vi "fgv_Sys Config.vi"(8 "error in (no error)":errorcluster, 10 "Function":T11, 11 "System Config in":T1={"XY Stage"={"COM port"="", "XY stage available"=FALSE}, "DAQ FPGA"={"Ref"=refnum, "Target"="RIO0", "Clock Freq (MHz) "=200.0, "input card type"=enum."AC Card", "Samples Wait after Trigger"=5080, "AOD fill"=4900, "StartupDelay"=0, "Slip Cycle (clock cycles)"=600000, "Add Cycle"=TRUE}, "Control system"={"Ethernet opened"=FALSE, "Ethernet Port"=3, "Ctrl FPGA available"=FALSE, "Ctrl FPGA Clock (MHz)"=240.0, "Ctrl system MAC address"="", "Control system.Network adapter name"="", "AOD 1 Amplitude"=0, "AOD 2 Amplitude"=0, "AOD 3 Amplitude"=0, "AOD 4 Amplitude"=0, "Data Time Interval (ns)"=0.0, "T0 (ns)"=0.0, "Ta (ns)"=0.0}, "Encoder"={"IP address"="224.0.1.103", "Port"=7000, "Encoder available"=FALSE, "Wheel radius (cm)"=16.0}, "DAQmx Chan"={"Pockels AO"="", "Hard shutter AO"="", "PMT AOs"="", "Power meter AI"=""}, "Computer MAC address"="", "Cam VidRec"={"DO flag-Video record"="", "DO flag-Trial start"="", "VidRec available"=FALSE}, "Externalise Triggers"=FALSE, "Laser wavelength (nm)"=920.0} {"Laser wavelength (nm)" min=800.0 max=1080.0 step=1.0; "Encoder"."Wheel radius (cm)" format="%#_13g"; "Control system"."Ctrl FPGA Clock (MHz)" min=80.0 max=500.0 step=1.0; "Control system"."Data Time Interval (ns)" min=0.0 max=2048.0 step=1.0; "Control system"."Ta (ns)" min=0.0 max=2048.0 step=1.0; "Control system"."T0 (ns)" min=0.0 max=2048.0 step=1.0; "Control system"."AOD 4 Amplitude" min=0 max=2048 step=1; "Control system"."AOD 3 Amplitude" min=0 max=2048 step=1; "Control system"."AOD 2 Amplitude" min=0 max=2048 step=1; "Control system"."AOD 1 Amplitude" min=0 max=2048 step=1}) -> (0 "error out":errorcluster, 3 "System Config out":T1={"XY Stage"={"COM port"="", "XY stage available"=FALSE}, "DAQ FPGA"={"Ref"=refnum, "Target"="RIO0", "Clock Freq (MHz) "=200.0, "input card type"=enum."AC Card", "Samples Wait after Trigger"=5080, "AOD fill"=4900, "StartupDelay"=0, "Slip Cycle (clock cycles)"=600000, "Add Cycle"=TRUE}, "Control system"={"Ethernet opened"=FALSE, "Ethernet Port"=3, "Ctrl FPGA available"=FALSE, "Ctrl FPGA Clock (MHz)"=240.0, "Ctrl system MAC address"="", "Control system.Network adapter name"="", "AOD 1 Amplitude"=0, "AOD 2 Amplitude"=0, "AOD 3 Amplitude"=0, "AOD 4 Amplitude"=0, "Data Time Interval (ns)"=0.0, "T0 (ns)"=0.0, "Ta (ns)"=0.0}, "Encoder"={"IP address"="224.0.1.103", "Port"=7000, "Encoder available"=FALSE, "Wheel radius (cm)"=16.0}, "DAQmx Chan"={"Pockels AO"="", "Hard shutter AO"="", "PMT AOs"="", "Power meter AI"=""}, "Computer MAC address"="", "Cam VidRec"={"DO flag-Video record"="", "DO flag-Trial start"="", "VidRec available"=FALSE}, "Externalise Triggers"=FALSE, "Laser wavelength (nm)"=920.0} {"Laser wavelength (nm)" min=800.0 max=1080.0 step=1.0; "Encoder"."Wheel radius (cm)" format="%#_13g"; "Control system"."Ctrl FPGA Clock (MHz)" min=80.0 max=500.0 step=1.0; "Control system"."Data Time Interval (ns)" min=0.0 max=2048.0 step=1.0; "Control system"."Ta (ns)" min=0.0 max=2048.0 step=1.0; "Control system"."T0 (ns)" min=0.0 max=2048.0 step=1.0; "Control system"."AOD 4 Amplitude" min=0 max=2048 step=1; "Control system"."AOD 3 Amplitude" min=0 max=2048 step=1; "Control system"."AOD 2 Amplitude" min=0 max=2048 step=1; "Control system"."AOD 1 Amplitude" min=0 max=2048 step=1})   [LabVIEW 2013]
uses:
  Typedefs/Sys Configuration.ctl
  Typedefs/XY Stage config cluster.ctl
  Typedefs/DAQ FPGA config cluster.ctl
  RIG-SPECIFIC FILES/FPGA Refs/FPGA Ref.ctl
  <vilib>/userdefined/High Color/nirio_resource_hc.ctl
  Typedefs/FPGA input type AC-DC.ctl
  Typedefs/CTRL system config cluster.ctl
  Typedefs/Encoder config cluster.ctl
  Typedefs/DAQmx physical channels cluster.ctl
  Typedefs/Cam VidRec HW config setup cluster.ctl
  Typedefs/HW config states enum.ctl
  Typedefs/Save-Load enum.ctl
panel:
  # "FUNCTIONAL GLOBAL"
  # "<--- The \"PMT AOs\" DAQmx string will always contain\n                       2 channels is this format: PXI1Slot4/ao2:3"
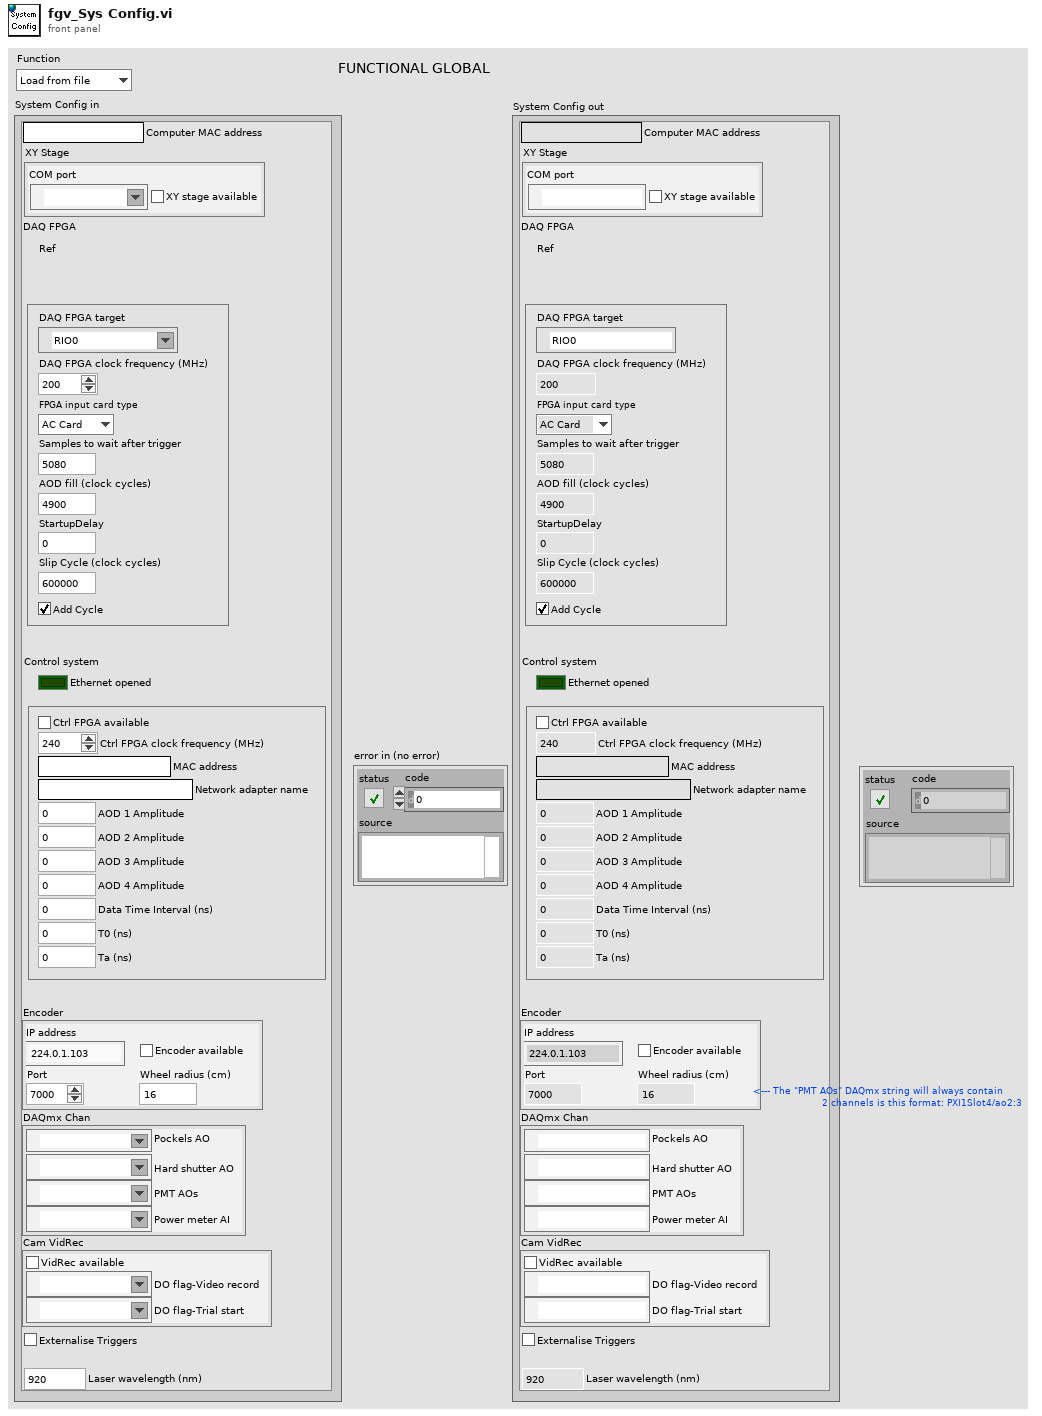
[diagram p1: front panel]
types:
  T1 = typedef "Sys Configuration.ctl" = cluster{"XY Stage":T2, "DAQ FPGA":T3, "Control system":T7, "Encoder":T8, "DAQmx Chan":T9, "Computer MAC address":string, "Cam VidRec":T10, "Externalise Triggers":bool, "Laser wavelength (nm)":dbl}
  T2 = typedef "XY Stage config cluster.ctl" = cluster{"COM port":refnum<visa-resource-name>, "XY stage available":bool}
  T3 = typedef "DAQ FPGA config cluster.ctl" = cluster{"Ref":T4, "Target":T5, "Clock Freq (MHz) ":dbl, "input card type":T6, "Samples Wait after Trigger":u16, "AOD fill":u16, "StartupDelay":i32, "Slip Cycle (clock cycles)":u32, "Add Cycle":bool}
  T4 = typedef "FPGA Ref.ctl" = refnum<k20>
  T5 = typedef "nirio_resource_hc.ctl" = tag
  T6 = typedef "FPGA input type AC-DC.ctl" = enum16{"AC Card", "DC Card"}
  T7 = typedef "CTRL system config cluster.ctl" = cluster{"Ethernet opened":bool, "Ethernet Port":u32, "Ctrl FPGA available":bool, "Ctrl FPGA Clock (MHz)":dbl, "Ctrl system MAC address":string, "Control system.Network adapter name":string, "AOD 1 Amplitude":i16, "AOD 2 Amplitude":i16, "AOD 3 Amplitude":i16, "AOD 4 Amplitude":i16, "Data Time Interval (ns)":dbl, "T0 (ns)":dbl, "Ta (ns)":dbl}
  T8 = typedef "Encoder config cluster.ctl" = cluster{"IP address":string, "Port":u16, "Encoder available":bool, "Wheel radius (cm)":dbl}
  T9 = typedef "DAQmx physical channels cluster.ctl" = cluster{"Pockels AO":tag, "Hard shutter AO":tag, "PMT AOs":tag, "Power meter AI":tag}
  T10 = typedef "Cam VidRec HW config setup cluster.ctl" = cluster{"DO flag-Video record":tag, "DO flag-Trial start":tag, "VidRec available":bool}
  T11 = typedef "HW config states enum.ctl" = enum16{"Load from file", "Save to file", "Write all", "Read all", "Write XY stage settings", "Write DAQ FPGA settings", "Write Control FPGA settings", "Write Phys Channels", "Clear", "Compare from file"}
  T12 = typedef "Save-Load enum.ctl" = enum16{"Save to file", "Load from file", "Compare from file"}
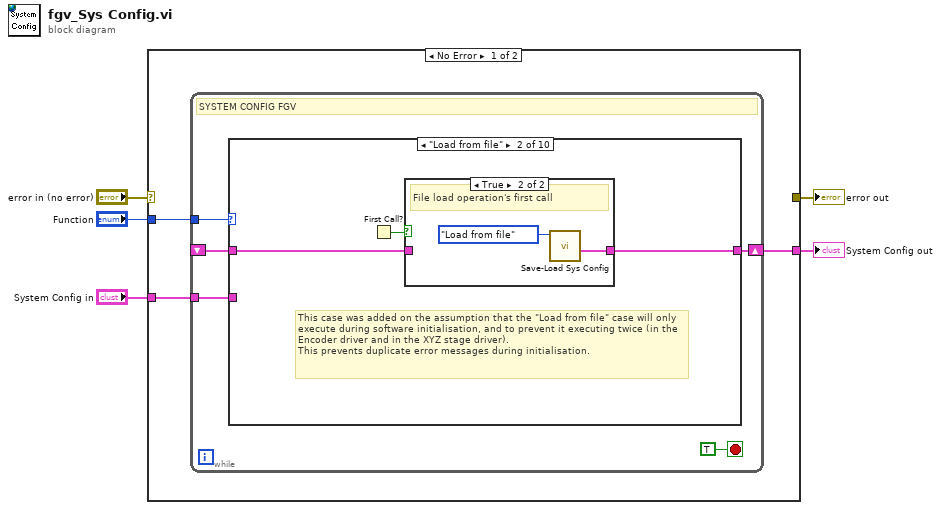
[diagram p0: block diagram]
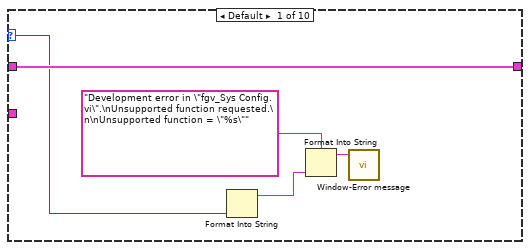
[diagram p2: hidden frame]
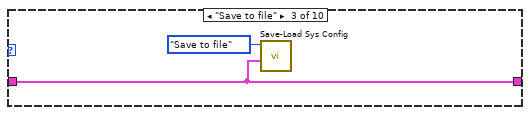
[diagram p4: hidden frame]
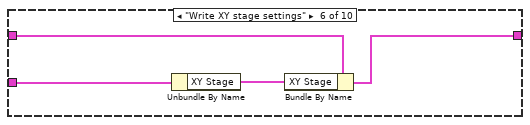
[diagram p7: hidden frame]
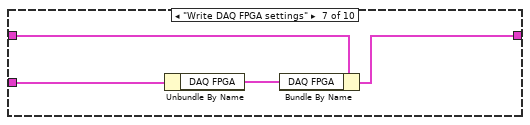
[diagram p8: hidden frame]
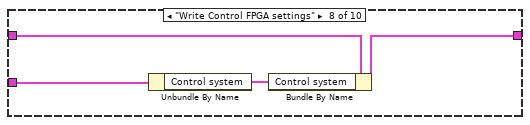
[diagram p9: hidden frame]
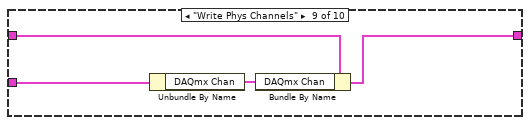
[diagram p10: hidden frame]
diagram:
  n1 = case shown="No Error" "error in (no error)" {
    selector: "error in (no error)" -> [_ w45]
    tunnel: [_ w45] -> w4
    tunnel: "Function" -> [w8 _]
    tunnel: "System Config in" -> [w7 _]
    tunnel: [w6 _] -> w1
    frame No Error {
      n2 = while {
        tunnel: w8 -> [w13]
        shift-right: [w11] -> w6
        shift-left: _ -> [w9]
        tunnel: w7 -> [w10]
        stop <- TRUE stop-if-true
        # "SYSTEM CONFIG FGV"
        n3 = case shown="\"Load from file\"" w13 {
          selector: w13 -> [w14 _ _ _ _ _ _ _ _ _]
          tunnel: [w15 w21 w26 w27 w28 w29 w33 w37 w41 _] -> w11
          tunnel: w10 -> [_ _ _ w27 _ w32 w36 w40 w44 _]
          tunnel: w9 -> [w15 w20 w26 _ w28 w31 w35 w39 w43 _]
          frame Default {
            n4 = Format Into String(w14) -> (resulting string=w17:string)  [unwired: 3 in, 1 out]
            n5 = Format Into String(format string="Development error in \"fgv_Sys Config.vi\".\nUnsupported function requested.\n\nUnsupported function = \"%s\"" ("Message"), w17) -> (resulting string=w16:string)  [unwired: 2 in, 1 out]
            n6 = call "Window-Error message.vi"("Message"=w16) -> ()  [unwired: 10 in, 1 out]
          }
          frame "Load from file" {
            # "This case was added on the assumption that the \"Load from file\" case will only execute during software initialisation, and to prevent it executing twice (in the Encoder driver and in the XYZ stage driver).\nThis prevents duplicate error messages during initialisation."
            n7 = First Call?() -> (First Call?: T/F=w19:bool)
            n8 = case shown="True" w19 {
              tunnel: [w22 w24] -> w21
              tunnel: w20 -> [w22 _]
              frame False {
                # "Already loaded"
              }
              frame True {
                # "File load operation's first call"
                n9 = call "Save-Load Sys Config.vi"("Function"=Save-Load_enum."Load from file") -> ("Loaded System config"=w24:T1)  [unwired: 9 in, 1 out]
              }
            }
          }
          frame "Save to file" {
            n10 = call "Save-Load Sys Config.vi"("System config to save"=w26, "Function"=Save-Load_enum."Save to file") -> ()  [unwired: 8 in, 2 out]
          }
          frame "Write all" {
          }
          frame "Read all" {
          }
          frame "Write XY stage settings" {
            n11 = Unbundle By Name(w32) -> ("XY Stage"=w30:T2)
            n12 = Bundle By Name(cluster=w31, "XY Stage"=w30) -> (w29:T1)
          }
          frame "Write DAQ FPGA settings" {
            n13 = Unbundle By Name(w36) -> ("DAQ FPGA"=w34:T3)
            n14 = Bundle By Name(cluster=w35, "DAQ FPGA"=w34) -> (w33:T1)
          }
          frame "Write Control FPGA settings" {
            n15 = Unbundle By Name(w40) -> ("Control system"=w38:T7)
            n16 = Bundle By Name(cluster=w39, "Control system"=w38) -> (w37:T1)
          }
          frame "Write Phys Channels" {
            n17 = Unbundle By Name(w44) -> ("DAQmx Chan"=w42:T9)
            n18 = Bundle By Name(cluster=w43, "DAQmx Chan"=w42) -> (w41:T1)
          }
          frame "Clear" {
          }
        }
      }
    }
    frame Error {
    }
  }
  "error out" <- w4
  "System Config out" <- w1
